vi "red buoyvi.vi"(0 "Image Src":T2, 1 "Cluster":cluster{"Max Radius":sgl, "Min Radius":sgl}={"Max Radius"=50.0, "Min Radius"=7.0}, 4 "error in (no error)":errorcluster) -> (6 "Image Out":T2(plugin-control), 7 "Circles Data (calibrated)":T1(array[cluster]), 8 "Nb Circles":i32, 9 "error out":errorcluster)   [LabVIEW 2009]
uses:
  <vilib>/vision/Image Controls.llb/IMAQ Image.ctl
  <vilib>/vision/NI_Vision_Development_Module.lvlib
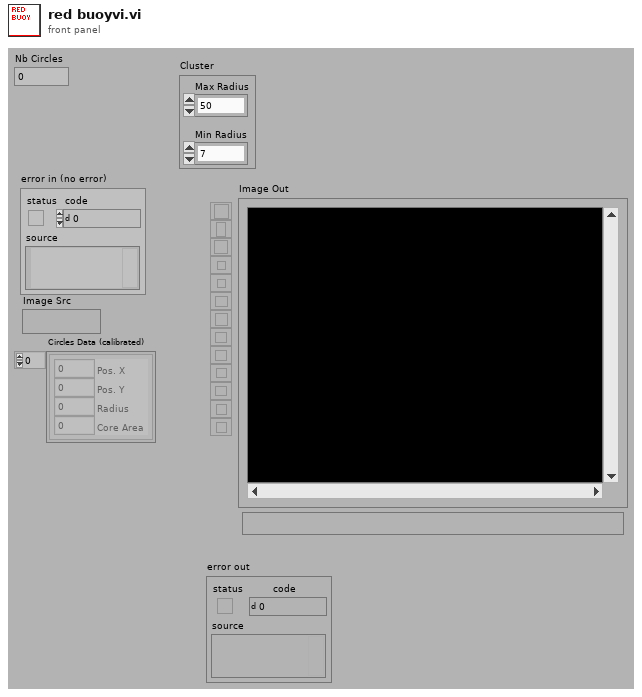
[diagram p1: front panel]
types:
  T1 = cluster{"Pos. X":i32, "Pos. Y":i32, "Radius":i32, "Core Area":i32}[]
  T2 = typedef "IMAQ Image.ctl" = refnum<image>
  T3 = enum32{"AutoM", "Close", "Dilate", "Erode", "Gradient", "Gradient out", "Gradient in", "Hit miss", "Open", "PClose", "POpen", "Thick", "Thin"}
  T4 = cluster{"Global Rectangle":i32[], "Contours":cluster{"ID":enum32{"External", "Internal"}, "Type":u32, "Coordinates":i32[]}[]}
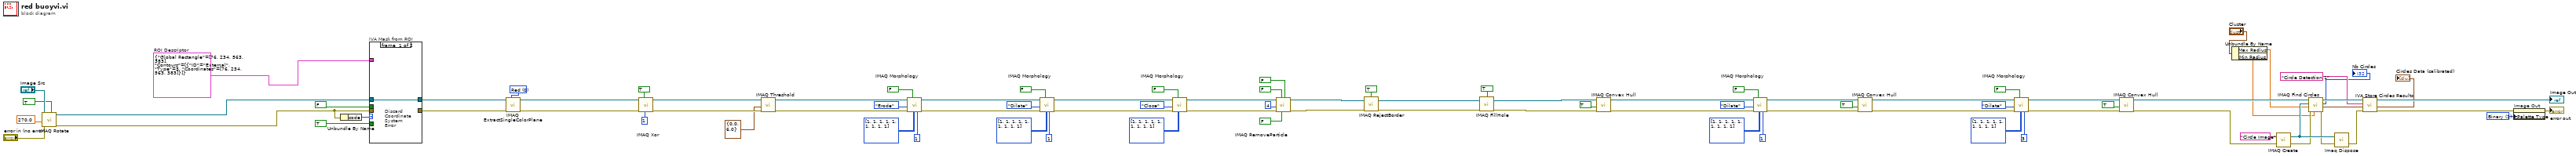
[diagram p0: block diagram]
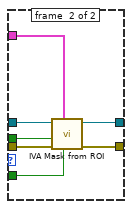
[diagram p2: hidden frame]
diagram:
  w7 = u32 1 items=["Grayscale", "Binary", "Gradient", "Rainbow", "Temperature", "User Defined"] ("Palette")
  w77 = 0 items=["Red", "Green", "Blue", "Hue", "Saturation", "Luminance", "Value", "Intensity"] ("Color Plane")
  w83 = T4 {"Global Rectangle"=[76, 234, 563, 383], "Contours"=[{"ID"=enum."External", "Type"=3, "Coordinates"=[76, 234, 563, 383]}]}  # ROI Descriptor
  n1 = call "IMAQ Rotate"("Maintain Size"=TRUE, "error in (no error)"="error in (no error)", "Angle (degrees)"=sgl 270.0, "Image Src"="Image Src") -> ("error out"=w86:errorcluster, "Image Dst Out"=w81:T2)  [unwired: 4 in, 2 out]
  n2 = Unbundle By Name(w86) -> ("code"=w78:i32)
  n3 = case "IVA Mask from ROI" shown="Default" w78 {
    tunnel: w83 -> [_ w96]
    tunnel: TRUE ("Shrink") -> [_ w95]
    tunnel: w81 -> [w89 w94]
    tunnel: w86 -> [_ w93]
    tunnel: [_ w92] -> w80
    tunnel: [w89 w91] -> w76
    tunnel: FALSE ("Out / In") -> [_ w90]
    frame #0 {
      # "Discard\nCoordinate\nSystem\nError"
    }
    frame #1 {
      n4 = call <vilib>:"IVA Mask from ROI.vi"("Shrink"=w95, "ROI Descriptor"=w96, "error in (no error)"=w93, "Out / In"=w90, "Image Src"=w94) -> ("error out"=w92:errorcluster, "Image Out"=w91:T2)  [unwired: 5 out]
    }
  }
  n5 = call "IMAQ ExtractSingleColorPlane"("Color Plane"=w77, "error in (no error)"=w80, "Image Src"=w76) -> ("error out"=w75:errorcluster, "Image Dst Out"=w72:T2)  [unwired: 1 in, 6 out]
  n6 = call "IMAQ Xor"("Constant"=1, "Xor/Xnor (Xor)"=TRUE, "error in (no error)"=w75, "Image Src A"=w72) -> ("error out"=w71:errorcluster, "Image Dst Out"=w69:T2)  [unwired: 2 in, 4 out]
  n7 = call "IMAQ Threshold"("error in (no error)"=w71, "Range"=cluster{"Lower value":sgl, "Upper value":sgl} {"Lower value"=0.0, "Upper value"=6.0}, "Image Src"=w69) -> ("error out"=w68:errorcluster, "Image Dst Out"=w63:T2)  [unwired: 3 in, 4 out]
  n8 = call "IMAQ Morphology"("Number of iterations (1)"=1, "Structuring Element"=i32[][] [[1, 1, 1], [1, 1, 1], [1, 1, 1]], "Square/Hexa (Square)"=FALSE, "error in (no error)"=w68, "Operation"=T3."Erode", "Image Src"=w63) -> ("error out"=w62:errorcluster, "Image Dst Out"=w57:T2)  [unwired: 1 in, 3 out]
  n9 = call "IMAQ Morphology"("Number of iterations (1)"=1, "Structuring Element"=i32[][] [[1, 1, 1], [1, 1, 1], [1, 1, 1]], "Square/Hexa (Square)"=FALSE, "error in (no error)"=w62, "Operation"=T3."Dilate", "Image Src"=w57) -> ("error out"=w56:errorcluster, "Image Dst Out"=w52:T2)  [unwired: 1 in, 3 out]
  n10 = call "IMAQ Morphology"("Structuring Element"=i32[][] [[1, 1, 1], [1, 1, 1], [1, 1, 1]], "Square/Hexa (Square)"=FALSE, "error in (no error)"=w56, "Operation"=T3."Close", "Image Src"=w52) -> ("error out"=w51:errorcluster, "Image Dst Out"=w46:T2)  [unwired: 2 in, 3 out]
  n11 = call "IMAQ RemoveParticle"("Connectivity 4/8 (8)"=FALSE, "Low Pass/High Pass (Low)"=FALSE, "Square/Hexa (Square)"=FALSE, "error in (no error)"=w51, "Number of Erosion"=4, "Image Src"=w46) -> ("error out"=w45:errorcluster, "Image Dst Out"=w43:T2)  [unwired: 1 in, 3 out]
  n12 = call "IMAQ RejectBorder"("error in (no error)"=w45, "Image Src"=w43, "Connectivity 4/8 (8)"=TRUE) -> ("error out"=w42:errorcluster, "Image Dst Out"=w40:T2)  [unwired: 1 in, 2 out]
  n13 = call "IMAQ FillHole"("error in (no error)"=w42, "Image Src"=w40, "Connectivity 4/8 (8)"=TRUE) -> ("error out"=w39:errorcluster, "Image Dst Out"=w38:T2)  [unwired: 1 in, 2 out]
  n14 = call "IMAQ Convex Hull"("error in (no error)"=w39, "Connectivity 4/8 (8)"=TRUE, "Image Src"=w38) -> ("error out"=w36:errorcluster, "Image Dst Out"=w31:T2)  [unwired: 1 in, 6 out]
  n15 = call "IMAQ Morphology"("Number of iterations (1)"=1, "Structuring Element"=i32[][] [[1, 1, 1], [1, 1, 1], [1, 1, 1]], "Square/Hexa (Square)"=FALSE, "error in (no error)"=w36, "Operation"=T3."Dilate", "Image Src"=w31) -> ("error out"=w30:errorcluster, "Image Dst Out"=w29:T2)  [unwired: 1 in, 3 out]
  n16 = call "IMAQ Convex Hull"("error in (no error)"=w30, "Connectivity 4/8 (8)"=TRUE, "Image Src"=w29) -> ("error out"=w27:errorcluster, "Image Dst Out"=w22:T2)  [unwired: 1 in, 6 out]
  n17 = call "IMAQ Morphology"("Number of iterations (1)"=3, "Structuring Element"=i32[][] [[1, 1, 1], [1, 1, 1], [1, 1, 1]], "Square/Hexa (Square)"=FALSE, "error in (no error)"=w27, "Operation"=T3."Dilate", "Image Src"=w22) -> ("error out"=w21:errorcluster, "Image Dst Out"=w20:T2)  [unwired: 1 in, 3 out]
  n18 = call "IMAQ Convex Hull"("error in (no error)"=w21, "Connectivity 4/8 (8)"=TRUE, "Image Src"=w20) -> ("error out"=w18:errorcluster, "Image Dst Out"=w11:T2)  [unwired: 1 in, 6 out]
  n19 = Unbundle By Name("Cluster") -> ("Max Radius"=w3:sgl, "Min Radius"=w2:sgl)
  n20 = call "IMAQ Create"("Image Name"="Circle Image", "error in (no error)"=w18) -> ("New Image"=w16:T2, "error out"=w15:errorcluster)  [unwired: 2 in, 1 out]
  n21 = call "IMAQ Find Circles"("Max Radius"=w2, "error in (no error)"=w15, "Min Radius"=w3, "Image Dst"=w16, "Image Src"=w11) -> ("error out"=w14:errorcluster, "Circles Data"=w9:T1, "Nb Circles"=→"Nb Circles":i32)  [unwired: 4 out]
  n22 = call "Imaq Dispose"("Image"=w16, "error in (no error)"=w14) -> ("error out"=w13:errorcluster)  [unwired: 1 in, 3 out]
  n23 = call <vilib>:"IVA Store Circles Results.vi"("error in (no error)"=w13, "Circles Data"=w9, "Step Name"="Circle Detection 1", "Image in"=w11) -> ("error out"=w12:errorcluster, "Circles Data (calibrated)"=→"Circles Data (calibrated)":T1, "Image dup"=→"Image Out":T2)  [unwired: 5 out]
  n24 = property on="Image Out" class="ImageControl"(error in=w12, "Palette:Palette Type"=w7) -> (error out=→"error out":errorcluster)  [unwired: 1 in, 1 out]
